vi "OpenCloseVI.vi"(3 "Task":enum16{"Open", "Close"}(ring), 4 "desired":T1, 5 "reference":refnum<vi>) -> ()   [LabVIEW 2014]
uses:
  SlideTypeDef.ctl
  LVPresent_Globals.vi
panel:
  out "Boolean":bool
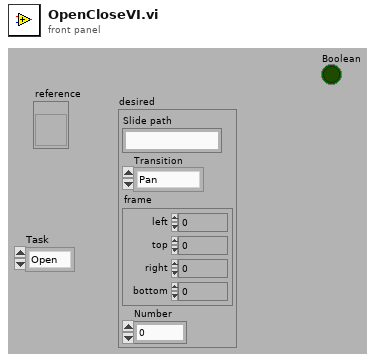
[diagram p1: front panel]
types:
  T1 = typedef "SlideTypeDef.ctl" = cluster{"Slide path":string, "Transition":enum16{"Pan", "Zoom-pan-zoom", "Zoom-wait-Zoom"}, "frame":cluster{"left":i16, "top":i16, "right":i16, "bottom":i16}, "Number":i32}
  T2 = enum32{"Bad", "Idle", "Run top level", "Running"}
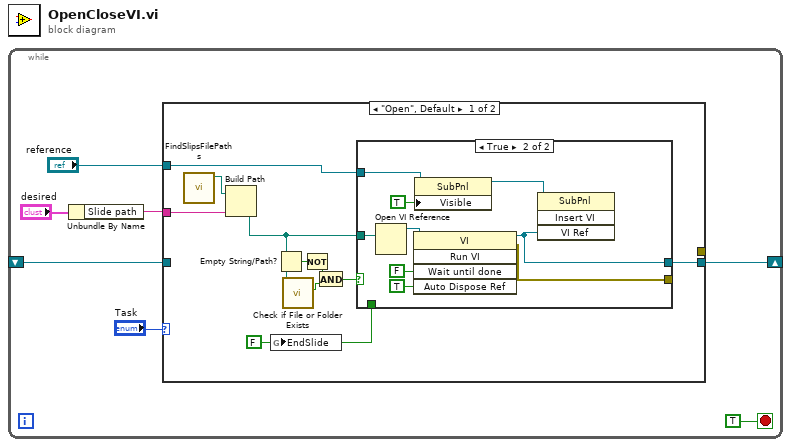
[diagram p0: block diagram]
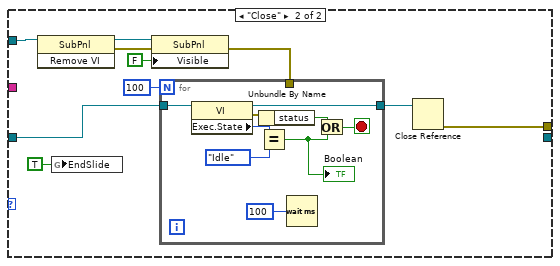
[diagram p3: hidden frame]
diagram:
  n1 = while {
    shift-right: [w4] -> _
    shift-left: _ -> [w3]
    stop <- TRUE stop-if-true
    n2 = Unbundle By Name("desired") -> ("Slide path"=w1:string)
    n3 = case shown="\"Open\", Default" "Task" {
      tunnel: "reference" -> [w13 w35]
      tunnel: [w12 _] -> w4
      tunnel: w3 -> [_ w31]
      tunnel: w1 -> [w10 _]
      tunnel: [_ w28] -> _
      frame "Open", Default {
        w8 = FALSE ("EndSlide")
        n4 = call "FindSlipsFilePaths.vi"() -> ("Slides"=w11:path)  [unwired: 2 in, 4 out]
        n5 = Build Path(base path=w11, name or relative path=w10) -> (appended path=w9:path)
        n6 = global write "LVPresent_Globals.vi" "EndSlide"(w8) -> ()
        n7 = Empty String/Path?(string/path=w9) -> (empty?=w14:bool)
        n8 = call <vilib>:"Check if File or Folder Exists.vi"("path"=w9) -> ("file or folder exists?"=w15:bool)  [unwired: 8 in, 2 out]
        n9 = Not(x=w14) -> (.not. x?=w16:bool)
        n10 = And(x=w16, y=w15) -> (x .and. y?=w17:bool)
        n11 = case shown="True" w17 {
          tunnel: w9 -> [_ w25]
          tunnel: w13 -> [_ w19]
          tunnel: [_ w24] -> w12
          tunnel: [_ w21] -> _
          tunnel: w8 -> [_ _]
          frame False {
          }
          frame True {
            n12 = Open VI Reference(vi path=w25) -> (vi reference=w26:refnum<vi>)  [unwired: 5 in, 1 out]
            n13 = invoke class="VI" method="Run VI"(reference=w26, "Wait until done"=FALSE ("Wait Until Done"), "Auto Dispose Ref"=TRUE ("Auto Dispose Reference")) -> (reference out=w24:refnum<vi>, error out=w21:errorcluster)  [unwired: 2 in, 3 out]
            n14 = property class="SubPnl"(reference=w19, "Visible"=TRUE) -> (reference out=w18:refnum<vi>)  [unwired: 1 in, 1 out]
            n15 = invoke on="Invoke Node" class="SubPnl" method="Insert VI"(reference=w18, "VI Ref"=w24) -> ()  [unwired: 2 in, 4 out]
          }
        }
      }
      frame "Close" {
        n16 = invoke on="Invoke Node" class="SubPnl" method="Remove VI"(reference=w35) -> (reference out=w33:refnum<vi>, error out=w32:errorcluster)  [unwired: 2 in, 1 out]
        n17 = global write "LVPresent_Globals.vi" "EndSlide"(TRUE ("EndSlide")) -> ()
        n18 = property class="SubPnl"(reference=w33, error in=w32, "Visible"=FALSE) -> (error out=w27:errorcluster)  [unwired: 1 out]
        n19 = for {
          N: 100 -> [_]
          tunnel: w31 -> [w45]
          tunnel: [w41] -> w29
          tunnel: w27 -> [_]
          stop <- w38 stop-if-true
          n20 = property class="VI"(reference=w45) -> (reference out=w41:refnum<vi>, error out=w40:errorcluster, "Exec.State"=w44:T2)  [unwired: 1 in]
          n21 = Unbundle By Name(w40) -> ("status"=w39:bool)
          n22 = Equal?(x=w44, y=T2."Idle" ("Execution:State")) -> (x = y?=w37:bool)
          "Boolean" <- w37
          n23 = Wait (ms)(milliseconds to wait=u32 100) -> ()  [unwired: 1 out]
          n24 = Or(x=w39, y=w37) -> (x .or. y?=w38:bool)
        }
        n25 = Close Reference(reference=w29) -> (error out=w28:errorcluster)  [unwired: 1 in]
      }
    }
  }
